vi "_Create Instrument Channel.vi"(4 "XON/XOFF (False)":bool, 6 "Baud Rate (921600 - USB)":u32=921600 min=300 max=115200 step=300, 7 "GPIB Board Add. (0)":u8 max=8 step=1, 8 "COM Port (1)":u16=1 min=1 max=9 step=1, 9 "GPIB Secondary Address (0)":u8 max=31 step=1, 10 "GPIB Primary Address (4)":u8=4 min=1 max=31 step=1, 11 "(F), T - GPIB, F - RS232":bool) -> (0 "Hardware Address":i32, 1 "Instrument Address":i16, 3 "Instrument Channel out":string="GPIB/0:4,0")   [LabVIEW 2014]
doc: "Builds the instrument channel handle (string) for an instrument connected over GPIB or RS-232. The default output string will be for a (USB) RS232 at Baud Rate of 921600.\n\nThis string should be passed in and out of the library vi's to control the specified insrument. Different handles should be used for controlling multiple instruments.\n\nThis will also initialize the RS-232 port to the speed specified, Which must be done manually if not using this vi."
panel:
  # "GPIB"
  # "RS-232"
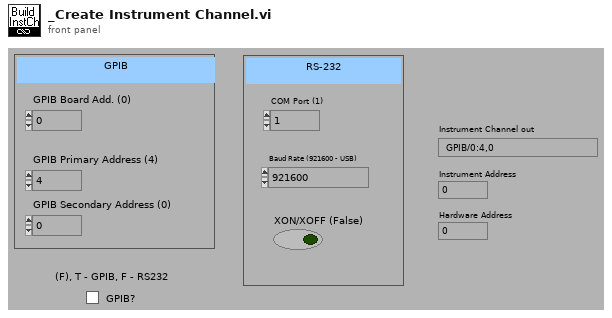
[diagram p1: front panel]
types:
  T1 = cluster{"input XON/XOFF":bool, "input HW Handshake":bool, "input alt HW HShk":bool, "output XON/XOFF":bool, "output HW Handshake":bool, "output alt HW HShk":bool, "XOFF byte ":u8, "XON byte":u8, "parity error byte":u16}
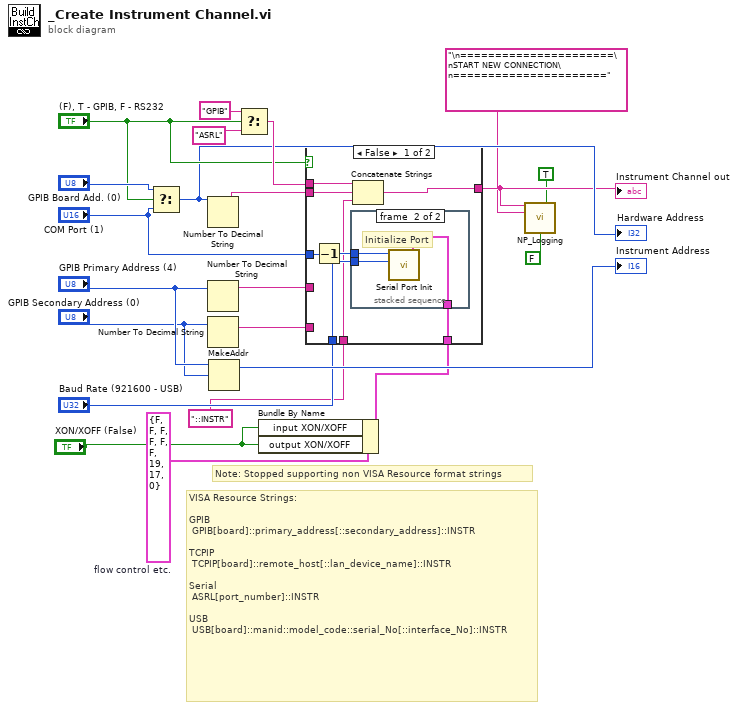
[diagram p0: block diagram]
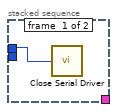
[diagram p2: hidden frame]
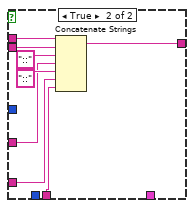
[diagram p3: hidden frame]
diagram:
  w3 = T1 {"input XON/XOFF"=FALSE, "input HW Handshake"=FALSE, "input alt HW HShk"=FALSE, "output XON/XOFF"=FALSE, "output HW Handshake"=FALSE, "output alt HW HShk"=FALSE, "XOFF byte "=19, "XON byte"=17, "parity error byte"=0}  # flow control etc.
  # "Note: Stopped supporting non VISA Resource format strings"
  # "VISA Resource Strings:\n\nGPIB\n GPIB[board]::primary_address[::secondary_address]::INSTR\n \nTCPIP\n TCPIP[board]::remote_host[::lan_device_name]::INSTR\n \nSerial\n ASRL[port_number]::INSTR\n \nUSB\n USB[board]::manid::model_code::serial_No[::interface_No]::INSTR"
  n1 = Select(t="GPIB Board Add. (0)", s="(F), T - GPIB, F - RS232", f="COM Port (1)") -> (s? t:f=w11:u16)
  "Hardware Address" <- w11
  n2 = Number To Decimal String(number=w11) -> (decimal integer string=w18:string)  [unwired: 1 in]
  n3 = Number To Decimal String(number="GPIB Primary Address (4)") -> (decimal integer string=w16:string)  [unwired: 1 in]
  n4 = Number To Decimal String(number="GPIB Secondary Address (0)") -> (decimal integer string=w15:string)  [unwired: 1 in]
  n5 = MakeAddr(3:"GPIB Secondary Address (0)", 4:"GPIB Primary Address (4)") -> (1:→"Instrument Address":i16)  [unwired: 1 in, 1 out]
  n6 = Select(t="GPIB", s="(F), T - GPIB, F - RS232", f="ASRL") -> (s? t:f=w19:string)
  n7 = Bundle By Name(cluster=w3, "input XON/XOFF"="XON/XOFF (False)", "output XON/XOFF"="XON/XOFF (False)") -> (w2:T1)
  n8 = case shown="False" "(F), T - GPIB, F - RS232" {
    tunnel: w18 -> [w30 w42]
    tunnel: w19 -> [w29 w41]
    tunnel: [w28 w40] -> w8
    tunnel: w16 -> [_ w37]
    tunnel: w15 -> [_ w36]
    tunnel: "COM Port (1)" -> [w27 _]
    tunnel: "Baud Rate (921600 - USB)" -> [w25 _]
    tunnel: "::INSTR" -> [w24 w35]
    tunnel: w2 -> [w23 _]
    frame False {
      n9 = Decrement(x=w27) -> (x-1=w26:u16)
      n10 = stacked-sequence {
        tunnel: w26 -> [w31 w34]
        tunnel: w25 -> [_ w33]
        tunnel: w23 -> [_ w32]
        frame #0 {
          n11 = call <vilib>:"Close Serial Driver.vi"("port number"=w31) -> ()  [unwired: 1 out]
        }
        frame #1 {
          # "Initialize Port"
          n12 = call <vilib>:"Serial Port Init.vi"("flow control etc."=w32, "baud rate"=w33, "port number"=w34) -> ()  [unwired: 4 in, 1 out]
        }
      }
      n13 = Concatenate Strings(w29, w30, w24) -> (w28:string)
    }
    frame True {
      n14 = Concatenate Strings(w41, w42, "::", w37, "::", w36, w35) -> (w40:string)
    }
  }
  "Instrument Channel out" <- w8
  n15 = call "NP_Logging.vi"("Instrument Channel"=w8, "Generic Strings"=TRUE, "String 1 {Write} (in)"="\n======================\nSTART NEW CONNECTION\n======================", "String 2 Enable (T)"=FALSE) -> ()  [unwired: 8 in, 4 out]
